vi "CheckDial.vi"(6 "error in":errorcluster, 9 "Knob in":refnum<class "Knob.lvclass">) -> (0 "error out":errorcluster, 3 "Knob out":refnum<class "Knob.lvclass">, 4 "Knob":bool, 5 "Size":i16)   [LabVIEW 2014, in "Knob.lvclass"]
uses:
  Knob.lvclass
  <vilib>/Utility/miscctls.llb/LVScalePositionTypeDef.ctl
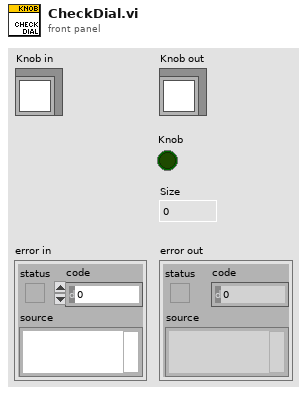
[diagram p1: front panel]
types:
  T1 = typedef "LVScalePositionTypeDef.ctl" = cluster{"Start":dbl, "Range":dbl}
  T2 = typedef "LVRangeTypeDef.ctl" = cluster{"Minimum":dbl, "Maximum":dbl, "Increment":dbl, "Minor Increment":dbl, "Start":dbl}
  T3 = typedef "imagedata.ctl" = cluster{"image type":i32, "image depth":i32, "image":u8[], "mask":u8[], "colors":u32[], "Rectangle":cluster{"left":i16, "top":i16, "right":i16, "bottom":i16}}
  T4 = cluster{"left":i16, "top":i16, "right":i16, "bottom":i16}
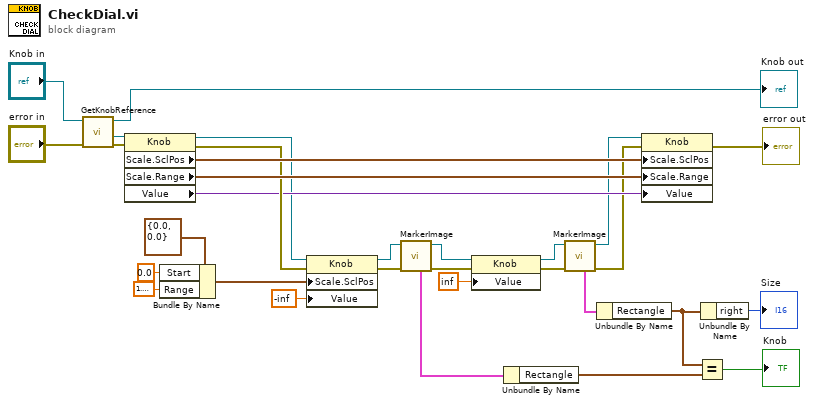
[diagram p0: block diagram]
diagram:
  n1 = call "GetKnobReference.vi"("error in"="error in", "Knob in"="Knob in") -> ("error out"=w5:errorcluster, "knob reference"=w6:refnum<vi>, "Knob out"=→"Knob out":refnum<class "Knob.lvclass">)  [unwired: 7 in]
  n2 = property on="Property Node" class="Knob"(reference=w6, error in=w5) -> (reference out=w22:refnum<vi>, error out=w29:errorcluster, "Scale.SclPos"=w31:T1, "Scale.Range"=w30:T2, "Value"=w28:variant)
  n3 = Bundle By Name(cluster=T1 {"Start"=0.0, "Range"=0.0} ("Scale.Scale Position"), "Start"=0.0, "Range"=1.5707963267948966) -> (w23:T1)
  n4 = property on="Property Node" class="Knob"(reference=w22, error in=w29, "Scale.SclPos"=w23, "Value"=-inf ("Knob 2")) -> (reference out=w20:refnum<vi>, error out=w21:errorcluster)
  n5 = call "MarkerImage.vi"("error in"=w21, "knob"=w20) -> ("error out"=w19:errorcluster, "knob reference out"=w18:refnum<vi>, "marker"=w12:T3)  [unwired: 5 in]
  n6 = property on="Property Node" class="Knob"(reference=w18, error in=w19, "Value"=inf ("Knob 2")) -> (reference out=w15:refnum<vi>, error out=w16:errorcluster)
  n7 = Unbundle By Name(w12) -> ("Rectangle"=w10:T4)
  n8 = call "MarkerImage.vi"("error in"=w16, "knob"=w15) -> ("error out"=w13:errorcluster, "knob reference out"=w14:refnum<vi>, "marker"=w11:T3)  [unwired: 5 in]
  n9 = Unbundle By Name(w11) -> ("Rectangle"=w8:T4)
  n10 = property on="Property Node" class="Knob"(reference=w14, error in=w13, "Scale.SclPos"=w31, "Scale.Range"=w30, "Value"=w28) -> (error out=→"error out":errorcluster)  [unwired: 1 out]
  n11 = Equal?(x=w8, y=w10) -> (x = y?=→"Knob":bool)
  n12 = Unbundle By Name(w8) -> ("right"=→"Size":i16)
